vi "New Execution.vi"(8 "error in (no error)":errorcluster) -> (0 "error out":errorcluster, 3 "Execution":refnum<data-value>)   [LabVIEW 2015, in "Execution.lvclass"]
uses:
  Execution.lvclass
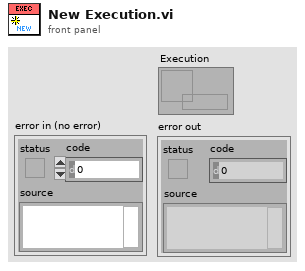
[diagram p1: front panel]
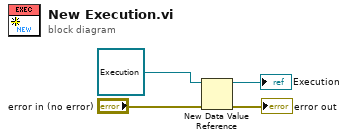
[diagram p0: block diagram]
diagram:
  n1 = New Data Value Reference(data value=refnum<class "Execution.lvclass"> refnum ("Socket.lvclass"), error in="error in (no error)") -> (data value reference=→"Execution":refnum<data-value>, error out=→"error out":errorcluster)
